vi "KE487_CommandsGlobal.vi"() -> ()   [LabVIEW 2019, in "KE487.lvclass"]
uses:
  KE487.lvclass
panel:
  in  "Keithley 487 GPIB Setup":T1={"Instrument name"="Keithley 487", "Command \"Reset\""="L0X", "Command \"Initialise\""="T8K0Q0W0Y0Z0G1F0B0C0P3R%dS1V0,1,%dO0U9H11X", "Command \"Arm\""="C2C0O1H11X", "Command \"SetVolts\""="V%3.2f,1,%dX", "Command \"Compliance?\""="U9X", "Command \"Standby\""="V0,0,0C1U9O0X\n", "Command \"Read Current\""="H11X"}
  # "T8: Multiple Trigger on Operate\nK0: Enable EOI and bus hold-off on X\nQ0: 175ms interval\nW0: Delay trigger 0sec\nY0: CR LF Terminator\nZ0: Disable relative\nG1: ASCII readings w/o prefix\nF0: Disable V/I ohms\nB0: Readings A/D\nC0: Disable zero check\nO0: Voltage source on standby\nU9: Send error status\nH11: Hit trigger key\n\nP3 (0-3) Filtering\nR0 (0-7) auto-range (1-7 fixed range)\nS1 (0-1) integration LineCycle\nV0,0 V0,1 voltage setting +voltage range\n,0 ,1 compliance"
  # "Set to zero volts\nclear compliance flag\nSwitch to standby"
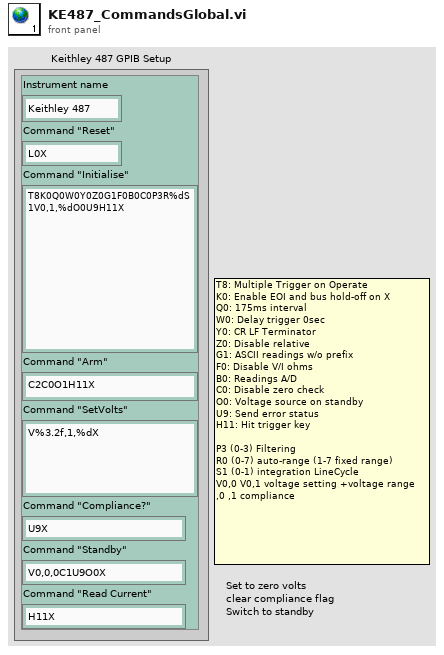
[diagram p1: front panel]
types:
  T1 = cluster{"Instrument name":string, "Command \"Reset\"":string, "Command \"Initialise\"":string, "Command \"Arm\"":string, "Command \"SetVolts\"":string, "Command \"Compliance?\"":string, "Command \"Standby\"":string, "Command \"Read Current\"":string}
diagram:
